vi "Creating New VI From Template.vi"() -> ()   [LabVIEW 2019]
doc: "Based on a user choice between addition and multiplication, this scripting VI creates a target VI that performs the chosen mathematical operation on an array of numbers. Instead of scripting the target VI one object at a time, this VI begins by copying template G code into the target VI and then making the necessary modifications. \n\nThe Detailed Help explains how this example illustrates a general procedure for creating a new VI from a pre-existing template VI."
panel:
  in  "Operation":u16(ring) items=["Add", "Multiply"]
  # "Select Help>>Show Context Help and move the cursor over the VI icon to display help for this VI."
  # "Before you start: Open the Detailed Help for this example to display the Creating a New VI from a Template Using VI Scripting topic in the  LabVIEW Help. That topic provides additional details about how this example illustrates the general procedure for creating a new VI from a pre-existing template VI.\n\nBased on a user choice between addition and multiplication, this scripting VI creates a target VI  that performs the chosen mathematical operation on an array of numbers. Instead of scripting the target VI one object at a time, this VI begins by copying template G code into the target VI and then making the necessary modifications.\n\nTurn on Execution Highlighting to observe the effects of each step in this scripting VI."
  # "Overview: Demonstrates the use of VI Scripting to programmatically replace a subVI on an existing block diagram.\nInstructions:\nRun the VI. A new VI based on a template is programmatically created, containing a subVI that performs the specified Operation, wired to a control and an indicator."
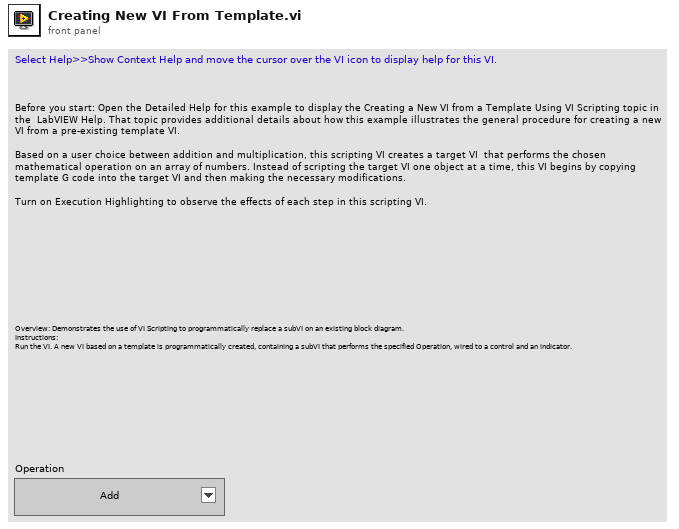
[diagram p1: front panel]
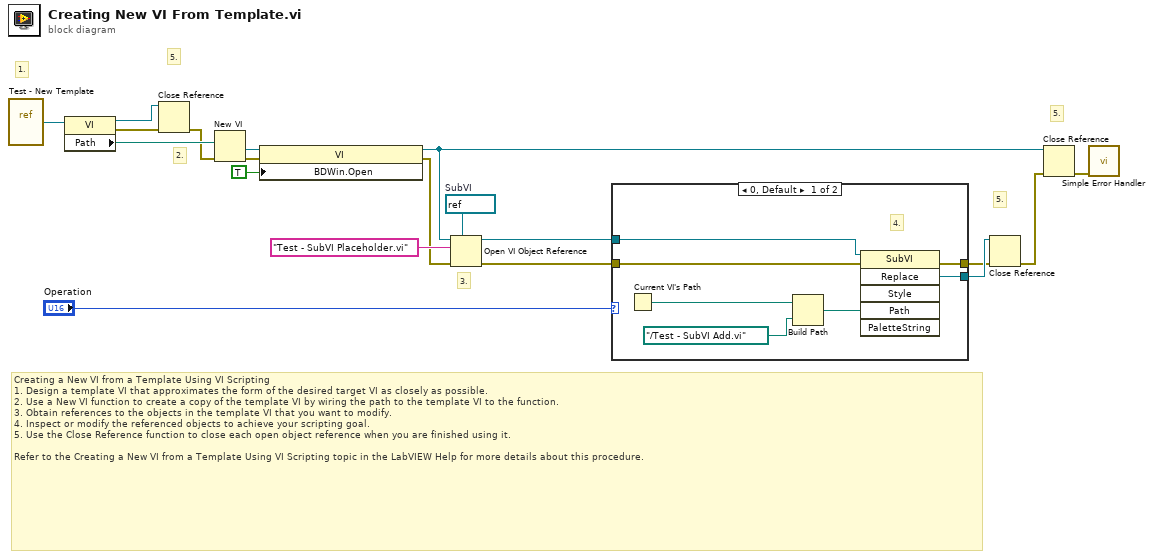
[diagram p0: block diagram]
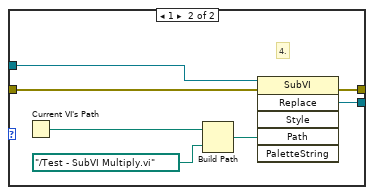
[diagram p2: hidden frame]
diagram:
  w19 = refnum<vi> refnum  # SubVI
  # "5."
  # "5."
  # "5."
  # "3."
  # "2."
  # "1."
  # "Creating a New VI from a Template Using VI Scripting\n1. Design a template VI that approximates the form of the desired target VI as closely as possible.\n2. Use a New VI function to create a copy of the template VI by wiring the path to the template VI to the function.\n3. Obtain references to the objects in the template VI that you want to modify.\n4. Inspect or modify the referenced objects to achieve your scripting goal.\n5. Use the Close Reference function to close each open object reference when you are finished using it.\n\nRefer to the Creating a New VI from a Template Using VI Scripting topic in the LabVIEW Help for more details about this procedure."
  n1 = vi-ref "Test - New Template.vi"() -> (w3:refnum<vi>)
  n2 = property on="Property Node" class="VI"(reference=w3) -> (reference out=w4:refnum<vi>, error out=w6:errorcluster, "Path"=w7:path)  [unwired: 1 in]
  n3 = Close Reference(reference=w4, error in (no error)=w6) -> (error out=w5:errorcluster)
  n4 = New VI(8:w5, 10:w7) -> (0:w10:errorcluster, 3:w12:refnum<vi>)  [unwired: 5 in]
  n5 = property on="Property Node" class="VI"(reference=w12, error in=w10, "BDWin.Open"=TRUE ("Front Panel Window:Open")) -> (reference out=w11:refnum<vi>, error out=w9:errorcluster)
  n6 = Open VI Object Reference(7:w19, 8:w9, 10:"Test - SubVI Placeholder.vi" ("name/order"), 11:w11) -> (0:w16:errorcluster, 3:w17:refnum<vi>)
  n7 = case shown="0, Default" "Operation" {
    tunnel: w17 -> [w26 w33]
    tunnel: [w25 w32] -> w15
    tunnel: w16 -> [w24 w31]
    tunnel: [w23 w30] -> w14
    frame 0, Default {
      # "4."
      n8 = Current VI's Path() -> (path=w20:path)
      n9 = Build Path(base path=w20, name or relative path=path "../Test - SubVI Add.vi" ("Path")) -> (appended path=w21:path)
      n10 = invoke on="Invoke Node" class="SubVI" method="Replace"(reference=w26, error in=w24, "Path"=w21) -> (error out=w23:errorcluster, "Replace"=w25:refnum<vi>)  [unwired: 3 in, 4 out]
    }
    frame 1 {
      # "4."
      n11 = Current VI's Path() -> (path=w27:path)
      n12 = Build Path(base path=w27, name or relative path=path "../Test - SubVI Multiply.vi" ("Path")) -> (appended path=w28:path)
      n13 = invoke on="Invoke Node" class="SubVI" method="Replace"(reference=w33, error in=w31, "Path"=w28) -> (error out=w30:errorcluster, "Replace"=w32:refnum<vi>)  [unwired: 3 in, 4 out]
    }
  }
  n14 = Close Reference(reference=w15, error in (no error)=w14) -> (error out=w13:errorcluster)
  n15 = Close Reference(reference=w11, error in (no error)=w13) -> (error out=w2:errorcluster)
  n16 = call <vilib>:"Simple Error Handler.vi"("error in (no error)"=w2) -> ()  [unwired: 4 in, 5 out]
